vi "Identify Tektronix.vi"(8 "error in":errorcluster, 11 "VISA resource name":refnum<visa-resource-name>) -> (0 "error out":errorcluster, 1 "Tektronix Driver.lvclass":refnum<class "Tektronix Driver.lvclass">, 3 "VISA resource name out":refnum<visa-resource-name>)   [LabVIEW 2020]
uses:
  Tektronix Driver/Tektronix Driver.lvclass
  Tektronix 4000 Driver/Tektronix 4000 Driver.lvclass
  C:/GitHub/NHMFL_Core/Libraries/Instruments/Tektronix/Tektronix Driver/Tektronix Driver.lvclass
  Tektronix 7000 Driver/Tektronix 7000 Driver.lvclass
  Tektronix MSO 6/Tektronix MSO 6 Driver.lvclass
  C:/GitHub/NHMFL_Core/Libraries/Instruments/Pulse Driver/Pulse Driver.lvclass
  C:/GitHub/NHMFL_Core/Libraries/Instruments/Instrument Driver/Instrument Driver.lvclass
  C:/GitHub/NHMFL_Core/Libraries/Instruments/Tektronix/Tektronix 4000 Driver/Tektronix 4000 Driver.lvclass
  C:/GitHub/NHMFL_Core/Libraries/Instruments/Tektronix/Tektronix 7000 Driver/Tektronix 7000 Driver.lvclass
  C:/GitHub/NHMFL_Core/Libraries/Instruments/Tektronix/Tektronix MSO 6/Tektronix MSO 6 Driver.lvclass
panel:
  out "data string out":string
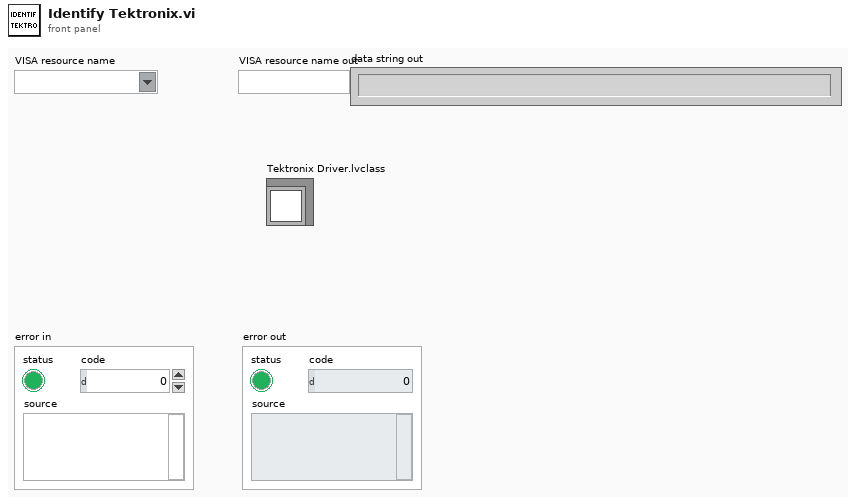
[diagram p1: front panel]
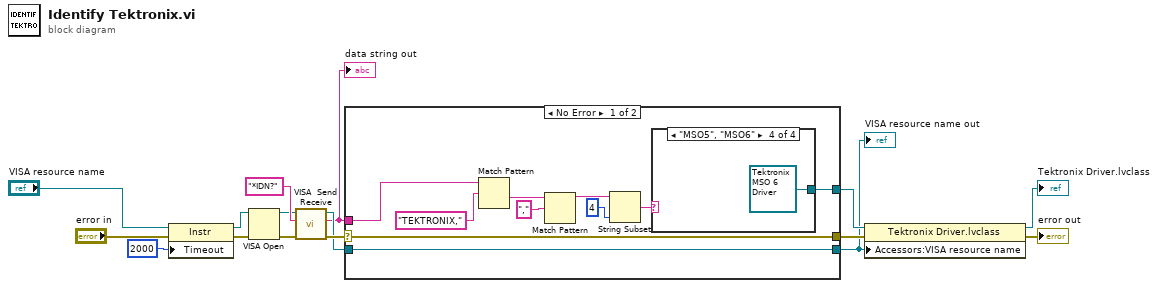
[diagram p0: block diagram]
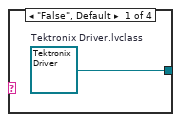
[diagram p2: hidden frame]
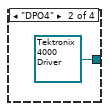
[diagram p3: hidden frame]
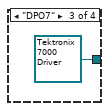
[diagram p4: hidden frame]
diagram:
  n1 = property class="Instr"(reference="VISA resource name", error in="error in", "Timeout"=u32 2000 ("General Settings:Timeout Value")) -> (reference out=w2:refnum<visa-resource-name>, error out=w4:errorcluster)
  n2 = VISA Open(error in (no error)=w4, VISA resource name=w2) -> (VISA resource name=w7:refnum<visa-resource-name>, error out=w6:errorcluster)  [unwired: 3 in]
  n3 = call "VISA  Send Receive.vi"("error in (no error)"=w6, "data string in"="*IDN?", "VISA Resource Name"=w7) -> ("error out"=w15:errorcluster, "data string out"=w12:string, "VISA Resource Name Out"=w14:refnum<visa-resource-name>)  [unwired: 6 in]
  "data string out" <- w12
  n4 = case shown="No Error" w15 {
    selector: w15 -> [w26 w32]
    tunnel: w14 -> [w25 w31]
    tunnel: [w22 _] -> w10
    tunnel: [w26 w32] -> w13
    tunnel: [w25 w31] -> w8
    tunnel: w12 -> [w24 _]
    frame No Error {
      n5 = Match Pattern(string=w24, regular expression="TEKTRONIX,") -> (after substring=w21:string)  [unwired: 1 in, 3 out]
      n6 = Match Pattern(string=w21, regular expression=",") -> (before substring=w19:string)  [unwired: 1 in, 3 out]
      n7 = String Subset(string=w19, length (rest)=4 ("length (rest)")) -> (substring=w18:string)  [unwired: 1 in]
      n8 = case shown="\"MSO5\", \"MSO6\"" w18 {
        tunnel: [w27 refnum<class "Tektronix 4000 Driver.lvclass"> refnum ("Tektronix 4000 Driver.lvclass") refnum<class "Tektronix 7000 Driver.lvclass"> refnum ("Tektronix 7000 Driver.lvclass") refnum<class "Tektronix MSO 6 Driver.lvclass"> refnum ("Tektronix MSO 6 Driver.lvclass")] -> w22
        frame "False", Default {
          w27 = refnum<class "Tektronix Driver.lvclass"> refnum  # Tektronix Driver.lvclass
        }
        frame "DPO4" {
        }
        frame "DPO7" {
        }
        frame "MSO5", "MSO6" {
        }
      }
    }
    frame Error {
    }
  }
  "VISA resource name out" <- w8
  n9 = property class="Tektronix Driver.lvclass"(reference=w10, error in=w13, "Accessors:VISA resource name"=w8) -> (reference out=→"Tektronix Driver.lvclass":refnum<class "Tektronix Driver.lvclass">, error out=→"error out":errorcluster)
